vi "AuMT8852B Default Single Payload Configuration.vi"(7 "Script (3)":i32=3, 8 "error in (no error)":errorcluster, 11 "VISA session":refnum<visa-resource-name>) -> (0 "error out":errorcluster, 2 "error code":i32, 3 "VISA session out":refnum<visa-resource-name>)   [LabVIEW 2017]
doc: "Anritsu MT8852B Bluetooth Tester\n\nReturns the system single-payload parameters to their default values.\n\nINPUTS\nScript - test script (3-10) to be reset to default single-payload parameters."
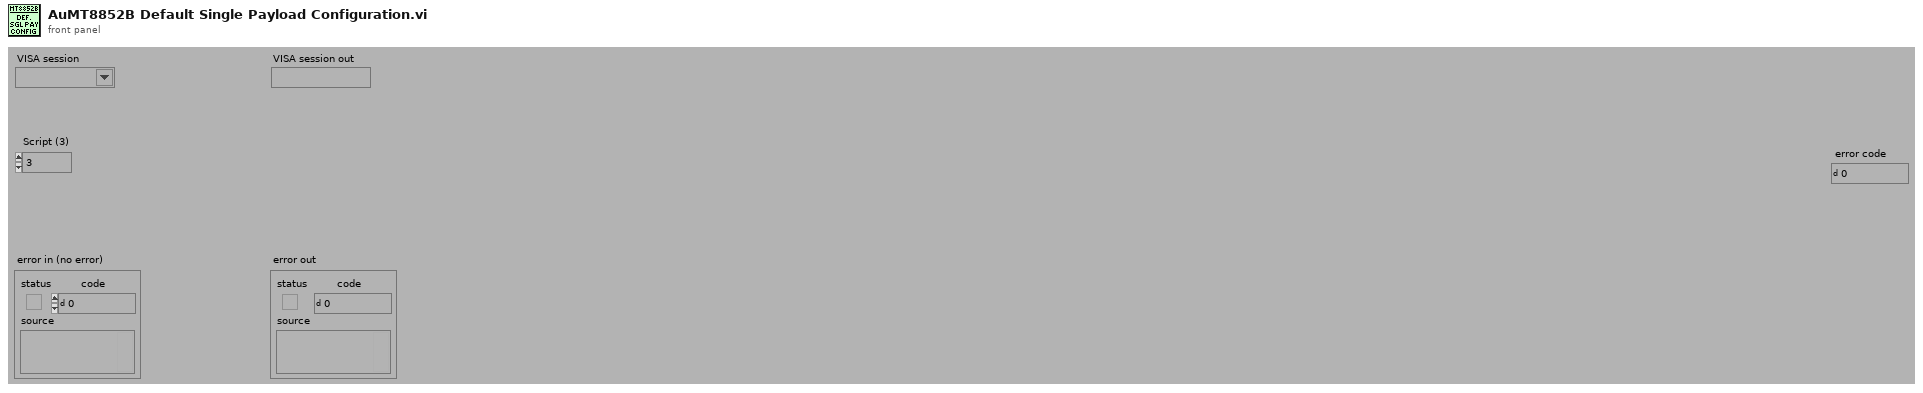
[diagram p1: front panel]
types:
  T1 = enum16{"Simulate", "Range check", "Cache", "Query instrument status"}
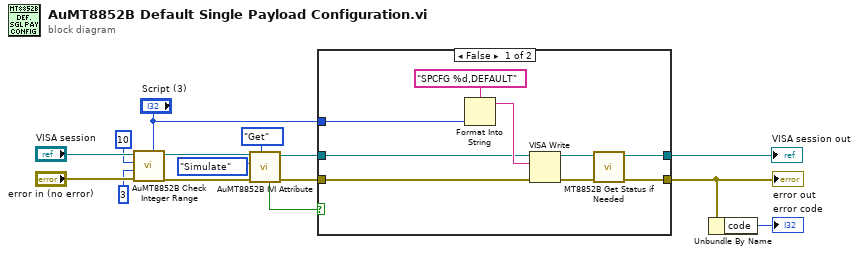
[diagram p0: block diagram]
diagram:
  n1 = call <instrlib>:"AuMT8852B Check Integer Range.vi"("Value (0)"="Script (3)", "error in (no error)"="error in (no error)", "Lower limit (-1)"=3, "Upper limit (1)"=10, "VISA session"="VISA session") -> ("error out"=w4:errorcluster, "VISA session out"=w5:refnum<visa-resource-name>)  [unwired: 5 in]
  n2 = call <instrlib>:"AuMT8852B IVI Attribute.vi"("Set/Get (Set)"=enum16{"Set", "Get"}."Get", "error in (no error)"=w4, "Flag (Simulate)"=T1."Simulate", "VISA session"=w5) -> ("error out"=w12:errorcluster, "VISA session out"=w13:refnum<visa-resource-name>, "Value out"=w10:bool)  [unwired: 5 in]
  n3 = case shown="False" w10 {
    tunnel: [w18 w25] -> w1
    tunnel: w13 -> [w22 w26]
    tunnel: w12 -> [w21 w25]
    tunnel: [w17 w26] -> w11
    tunnel: "Script (3)" -> [w16 _]
    frame False {
      n4 = Format Into String(format string="SPCFG %d,DEFAULT" ("Format String"), w16) -> (resulting string=w23:string)  [unwired: 2 in, 1 out]
      n5 = VISA Write(VISA resource name=w22, write buffer=w23, error in (no error)=w21) -> (VISA resource name out=w20:refnum<visa-resource-name>, error out=w19:errorcluster)  [unwired: 1 out]
      n6 = call <instrlib>:"MT8852B Get Status if Needed.vi"("error in (no error)"=w19, "VISA session"=w20) -> ("error out"=w18:errorcluster, "VISA session out"=w17:refnum<visa-resource-name>)  [unwired: 8 in]
    }
    frame True {
    }
  }
  "VISA session out" <- w11
  "error out" <- w1
  n7 = Unbundle By Name(w1) -> ("code"=→"error code":i32)
